vi "Process.vi"(1 "Process Name":string="Winword") -> (0 "Process find":bool)   [LabVIEW 2015]
uses:
  KERNEL32.DLL
  psapi.dll
panel:
  out "process handle":u32
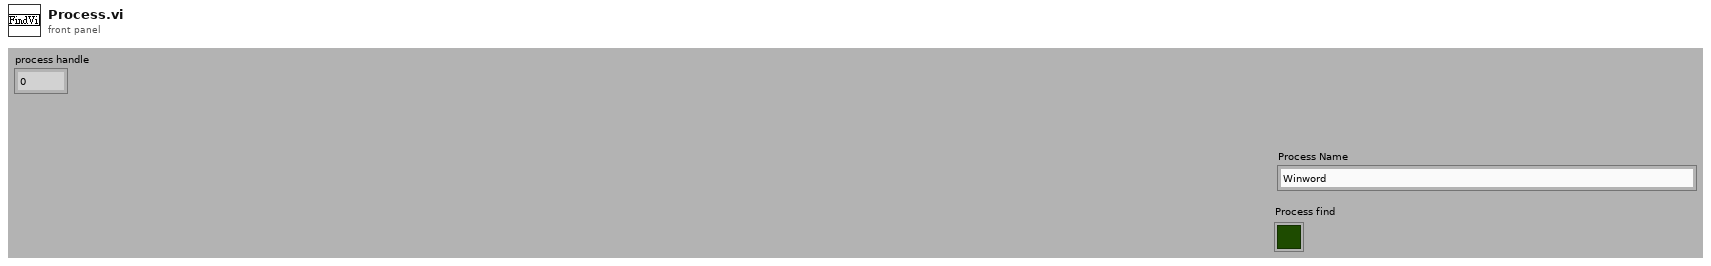
[diagram p1: front panel]
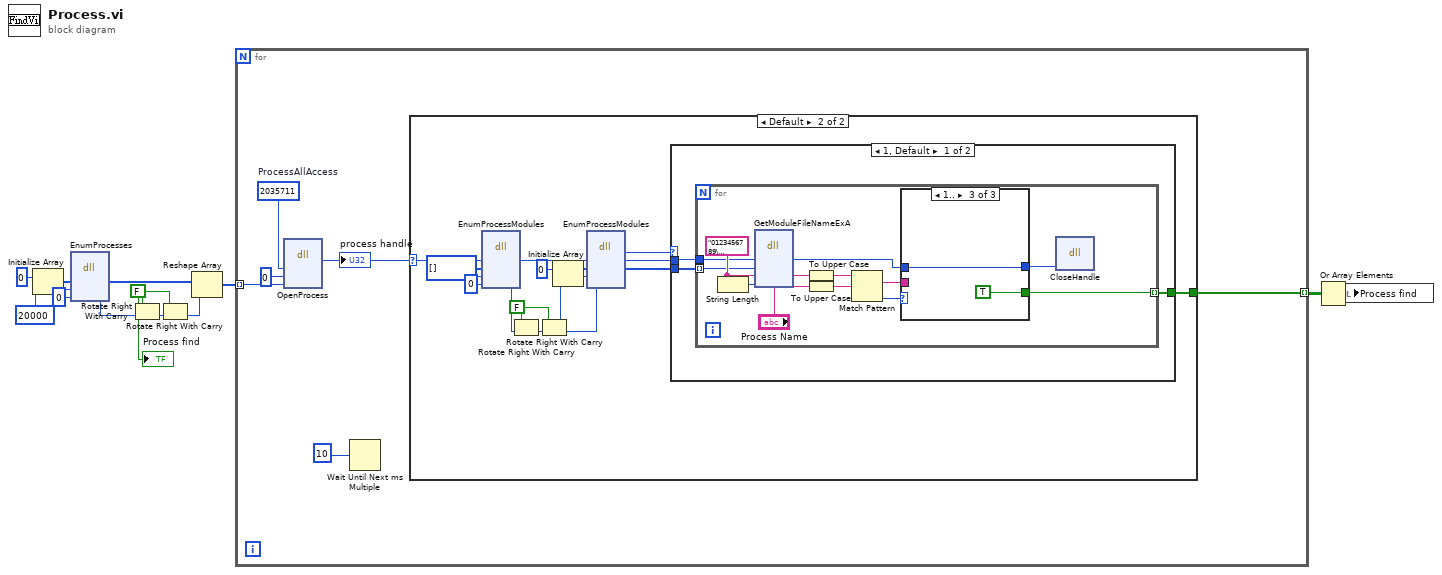
[diagram p0: block diagram]
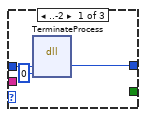
[diagram p3: hidden frame]
diagram:
  w3 = FALSE ("carry")
  w10 = 20000
  n1 = Initialize Array(u32 0, w10) -> (w11:u32[])
  n2 = dll-call lib="psapi.dll" fn="EnumProcesses"("lpidProcess"=w11, "cb"=w10, "cbNeeded"=u32 0) -> ("lpidProcess"=w7:u32[], "cbNeeded"=w8:u32)  [unwired: 5 in, 2 out]
  n3 = Rotate Right With Carry(2:w8, 3:w3) -> (0:w5:u32)  [unwired: 1 out]
  n4 = Rotate Right With Carry(2:w5, 3:w3) -> (0:w4:u32)  [unwired: 1 out]
  n5 = Reshape Array(w7, w4) -> (w6:u32[])
  n6 = for {
    tunnel: w6 -> [w16] mode=indexing
    tunnel: [w13] -> w1 mode=indexing
    w14 = 2035711  # ProcessAllAccess
    n7 = dll-call lib="KERNEL32.DLL" fn="OpenProcess"("dwDesiredAccessas"=w14, "bInheritHandle"=0, "dwProcId"=w16) -> (w15:u32)  [unwired: 6 in, 2 out]
    "process handle" <- w15
    n8 = Wait Until Next ms Multiple(millisecond multiple=10) -> ()  [unwired: 1 out]
    n9 = case shown="Default" w15 {
      selector: w15 -> [_ w32]
      tunnel: [_ w19] -> w13
      frame 0 {
      }
      frame Default {
        w28 = FALSE ("carry")
        w31 = 0 ("cbNeeded")
        n10 = dll-call lib="psapi.dll" fn="EnumProcessModules"("hProcesses"=w32, "lphModule"=u32[] [], "cb"=w31, "cbNeeded"=w31) -> ("hProcesses"=w23:u32, "cbNeeded"=w26:i32)  [unwired: 6 in, 2 out]
        n11 = Rotate Right With Carry(2:w26, 3:w28) -> (0:w27:i32)  [unwired: 1 out]
        n12 = Rotate Right With Carry(2:w27, 3:w28) -> (0:w24:i32)  [unwired: 1 out]
        n13 = Initialize Array(u32 0, w24) -> (w25:u32[])
        n14 = dll-call lib="psapi.dll" fn="EnumProcessModules"("hProcesses"=w23, "lphModule"=w25, "cb"=w24, "cbNeeded"=w24) -> (w22:u32, "hProcesses"=w21:u32, "lphModule"=w20:u32[])  [unwired: 5 in, 2 out]
        n15 = case shown="1, Default" w22 {
          tunnel: w21 -> [w35 _]
          tunnel: w20 -> [w34 _]
          tunnel: [w33 _] -> w19
          frame 1, Default {
            n16 = for {
              tunnel: w35 -> [w46]
              tunnel: w34 -> [w45] mode=indexing
              tunnel: [w39] -> w33 mode=indexing
              w47 = "0123456789\n0123456789\n0123456789\n0123456789\n0123456789\n01234567890123456789\n0123456789\n0123456789\n0123456789\n0123456789\n01234567890123456789\n0123456789\n0123456789\n0123456789\n0123456789\n01234567890123456789\n0123456789\n0123456789\n0123456789\n0123456789\n01234567890123456789\n0123456789\n0123456789\n0123456789\n0123456789\n01234567890123456789\n0123456789\n0123456789\n0123456789\n0123456789\n0123456789"
              n17 = String Length(string=w47) -> (length=w48:i32)
              n18 = dll-call lib="psapi.dll" fn="GetModuleFileNameExA"("hProcess"=w46, "hModule"=w45, "ModuleName"=w47, "nSize"=w48) -> ("hProcess"=w41:u32, "ModuleName"=w40:string)  [unwired: 6 in, 2 out]
              n19 = To Upper Case(1:w40) -> (0:w37:string)
              n20 = To Upper Case(1:"Process Name") -> (0:w36:string)
              n21 = Match Pattern(string=w37, regular expression=w36) -> (match substring=w42:string, offset past match=w38:i32)  [unwired: 1 in, 2 out]
              n22 = case shown="1.." w38 {
                tunnel: w41 -> [w50 w52 w54]
                tunnel: [w49 w52 w54] -> w43
                tunnel: w42 -> [_ _ _]
                tunnel: [_ _ TRUE] -> w39
                frame ..-2 {
                  n23 = dll-call lib="KERNEL32.DLL" fn="TerminateProcess"("hProcess"=w50, "uExitCode"=0) -> ("hProcess"=w49:u32)  [unwired: 5 in, 2 out]
                }
                frame -1, Default {
                }
                frame 1.. {
                }
              }
              n24 = dll-call lib="KERNEL32.DLL" fn="CloseHandle"("Handle"=w43) -> ()  [unwired: 5 in, 2 out]
            }
          }
          frame 0 {
          }
        }
      }
    }
  }
  n25 = Or Array Elements(Boolean array=w1) -> (logical OR=w2:bool)
  n26 = local write "Process find"(w2) -> ()
  "Process find" <- w3
